vi "automatic_recipe_write.vi"(7 "references":T2, 8 "error in (no error)":errorcluster, 10 "transition":string, 11 "recipe []":T1[](array[typedef])=[{"step"="", "data"=variant}]) -> (0 "error out":errorcluster)   [LabVIEW 2015, in "lv-recipe-machine.lvlib"]
uses:
  lv-recipe-machine.lvlib
  _controls/references.ctl
  _controls/input.ctl
  _controls/input_command.ctl
  _controls/output.ctl
  _controls/data.ctl
  _controls/configuration.ctl
  _controls/recipe_data.ctl
  _controls/mode.ctl
  _controls/manual_state.ctl
  _controls/automatic_state.ctl
  _controls/recipe_step.ctl
  _controls/change.ctl
  _controls/status.ctl
  _controls/transition.ctl
  _controls/error.ctl
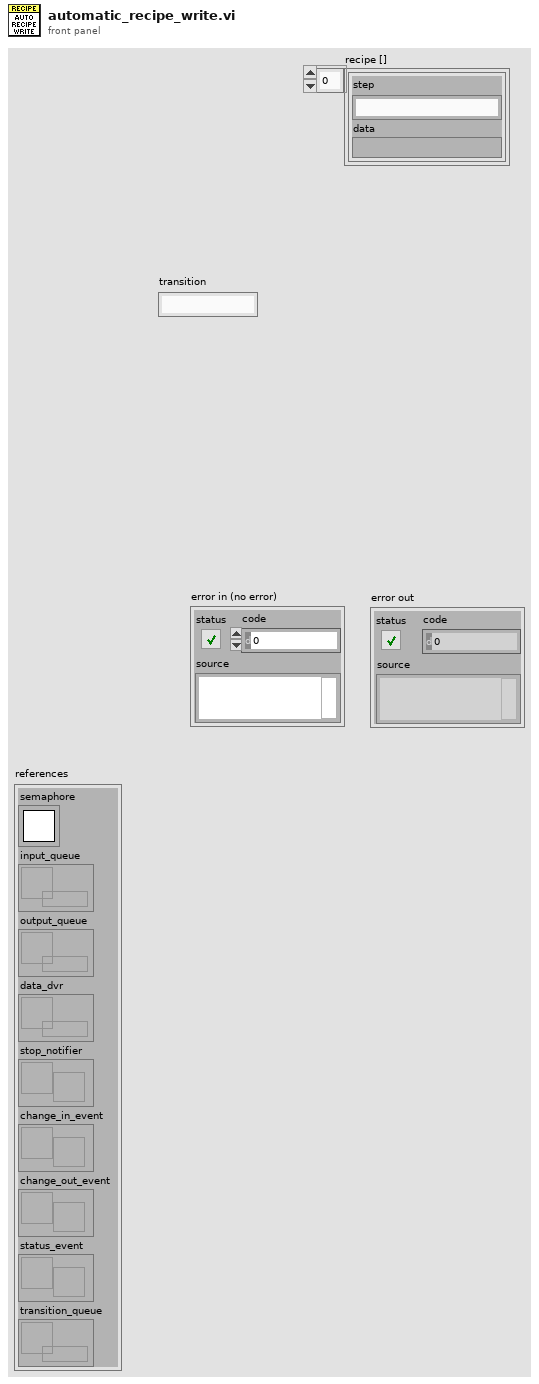
[diagram p1: front panel]
types:
  T1 = typedef "lv-recipe-machine.lvlib/recipe_step.ctl" = cluster{"step":string, "data":variant}
  T2 = typedef "lv-recipe-machine.lvlib/references.ctl" = cluster{"semaphore":T3, "input_queue":refnum<queue>, "output_queue":refnum<queue>, "data_dvr":refnum<data-value>, "stop_notifier":refnum<notifier>, "change_in_event":refnum<user-event>, "change_out_event":refnum<user-event>, "status_event":refnum<user-event>, "transition_queue":refnum<queue>}
  T3 = typedef "Semaphore RefNum" = refnum<k1>
  T4 = typedef "lv-recipe-machine.lvlib/error.ctl" = enum16{"<error>", "bad_command", "command_queue_timeout", "stop_notifier_timeout", "die_command_timeout", "not_in_manual_mode", "not_in_automatic_mode", "not_in_automatic_idle", "not_in_automatic_running", "not_in_automatic_paused", "automatic_step_not_found", "manual_action_not_found", "automatic_not_transition_vi", "transition_step_not_found", "unsupported_vi_type", "<null>"}
  T5 = typedef "lv-recipe-machine.lvlib/data.ctl" = cluster{"configuration":T6, "working":cluster{"recipe_data":T7}}
  T6 = typedef "lv-recipe-machine.lvlib/configuration.ctl" = cluster{"max_processes":i32}
  T7 = typedef "lv-recipe-machine.lvlib/recipe_data.ctl" = cluster{"mode":T8, "manual_state":T9, "automatic_state":T10, "previous_automatic_state":T10, "error":errorcluster, "manual":cluster{"step_action":string, "data":variant, "actions":variant}, "automatic":cluster{"data":variant, "steps":variant, "criteria":variant, "transition":string, "index":i32, "recipe []":T1[]}}
  T8 = typedef "lv-recipe-machine.lvlib/mode.ctl" = enum16{"<mode>", "manual", "automatic", "<null>"}
  T9 = typedef "lv-recipe-machine.lvlib/manual_state.ctl" = enum16{"<manual_state>", "failed", "action", "running", "idle", "<null>"}
  T10 = typedef "lv-recipe-machine.lvlib/automatic_state.ctl" = enum16{"<automatic_state>", "failed", "idle", "running", "paused", "stopped", "<null>"}
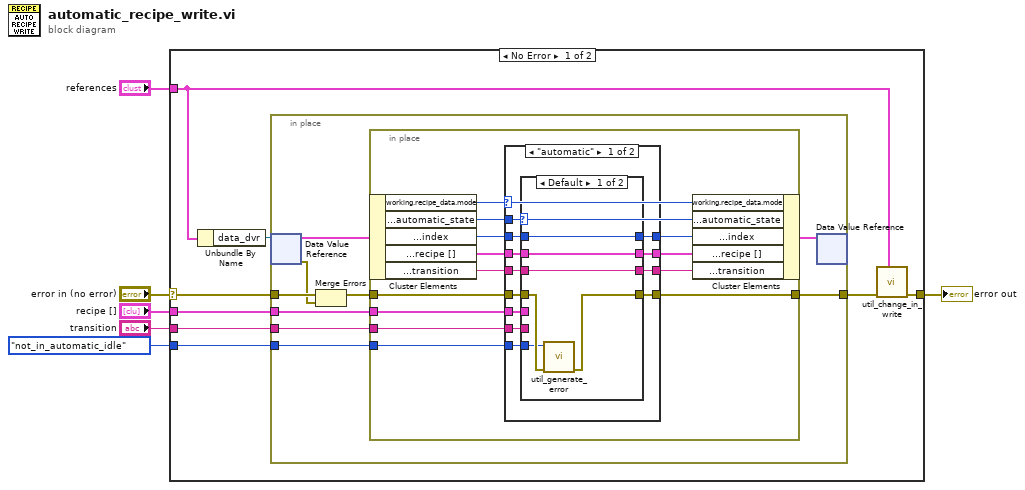
[diagram p0: block diagram]
diagram:
  n1 = case shown="No Error" "error in (no error)" {
    selector: "error in (no error)" -> [w13 w61]
    tunnel: [w11 w61] -> w4
    tunnel: "references" -> [w12 _]
    tunnel: "recipe []" -> [w10 _]
    tunnel: error."not_in_automatic_idle" ("error") -> [w8 _]
    tunnel: "transition" -> [w7 _]
    frame No Error {
      n2 = Unbundle By Name(w12) -> ("data_dvr"=w14:refnum<data-value>)
      n3 = in-place {
        in-place-border: w13 -> [w23]
        in-place-border: w10 -> [w18]
        in-place-border: [w17] -> w9
        in-place-border: w8 -> [w16]
        in-place-border: w7 -> [w15]
        n4 = in-place-dvr #1(w14) -> (w21:T5, w22:errorcluster)
        n5 = Merge Errors(w23, w22) -> (w19:errorcluster)
        n6 = in-place {
          in-place-border: w19 -> [w31]
          in-place-border: w18 -> [w32]
          in-place-border: [w30] -> w17
          in-place-border: w16 -> [w29]
          in-place-border: w15 -> [w26]
          n7 = in-place-cluster #2(w21) -> ("working.recipe_data.mode"=w34:T8, "working.recipe_data.automatic_state"=w33:T10, "working.recipe_data.automatic.index"=w28:i32, "working.recipe_data.automatic.recipe []"=w36:T1[], "working.recipe_data.automatic.transition"=w25:string)
          n8 = case shown="\"automatic\"" w34 {
            tunnel: w33 -> [w48 _]
            tunnel: w36 -> [w46 _]
            tunnel: [w45 w59] -> w35
            tunnel: w32 -> [w47 w59]
            tunnel: w31 -> [w44 w60]
            tunnel: [w43 w60] -> w30
            tunnel: w29 -> [w42 _]
            tunnel: w28 -> [w41 _]
            tunnel: [w40 _] -> w27
            tunnel: w26 -> [w39 w58]
            tunnel: w25 -> [w38 _]
            tunnel: [w37 w58] -> w24
            frame "automatic" {
              n9 = case shown="Default" w48 {
                tunnel: w47 -> [_ w56]
                tunnel: w46 -> [w52 _]
                tunnel: [w52 w56] -> w45
                tunnel: w44 -> [w54 w57]
                tunnel: [w53 w57] -> w43
                tunnel: w42 -> [w51 _]
                tunnel: w41 -> [w50 _]
                tunnel: [w50 _] -> w40
                tunnel: w39 -> [_ w55]
                tunnel: w38 -> [w49 _]
                tunnel: [w49 w55] -> w37
                frame Default {
                  n10 = call "util_generate_error.vi"("error in (no error)"=w54, "error"=w51) -> ("error out"=w53:errorcluster)  [unwired: 9 in]
                }
                frame "idle" {
                }
              }
            }
            frame Default {
            }
          }
          n11 = in-place-cluster #2("working.recipe_data.mode"=w34, "working.recipe_data.automatic_state"=w33, "working.recipe_data.automatic.index"=w27, "working.recipe_data.automatic.recipe []"=w35, "working.recipe_data.automatic.transition"=w24) -> (w20:T5)
        }
        n12 = in-place-dvr #1(w20) -> ()  [unwired: 2 out]
      }
      n13 = call "util_change_in_write.vi"("references"=w12, "error in (no error)"=w9) -> ("error out"=w11:errorcluster)  [unwired: 9 in]
    }
    frame Error {
    }
  }
  "error out" <- w4
